vi "PH_uOPA_DelayController.PC _Settings.vi"(0 "VI in":refnum<vi>, 1 "serviceName":string, 2 "Axis Settings":T1={"Sign change"=FALSE, "Width"=0.0, "Calibration"=0.0, "Unit"="Steps", "Motor Type"=enum."Unspecific", "Unit Width"="", "Unit CF"=""}, 4 "no link":bool, 5 "error in (no error)":errorcluster) -> (14 "VI out":refnum<vi>, 19 "error out":errorcluster)   [LabVIEW 2014, in "PH_uOPA_DelayController.lvlib"]
uses:
  PH_uOPA_DelayController.lvlib
  PH_Basics/PH_Stepmotor_BaseClass/PH_Stepmotor_BaseClass.Axis Settings.ctl
  PH_Basics/PH_Stepmotor_BaseClass/PH_Stepmotor_BaseClass.Motor Type.ctl
  PH_Basics/PH_AxisGUI_BaseClass/PH_AxisGUI_BaseClass.lvlib
  PH_Basics/PH_Stepmotor_BaseClass/PH_Stepmotor_BaseClass.lvlib
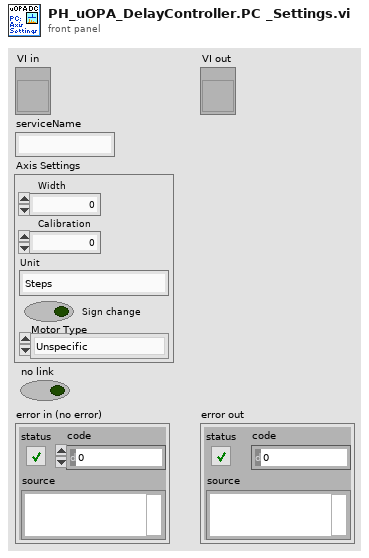
[diagram p1: front panel]
types:
  T1 = typedef "PH_Stepmotor_BaseClass.lvlib/PH_Stepmotor_BaseClass.Axis Settings.ctl" = cluster{"Sign change":bool, "Width":dbl, "Calibration":dbl, "Unit":string, "Motor Type":T2, "Unit Width":string, "Unit CF":string}
  T2 = typedef "PH_Stepmotor_BaseClass.lvlib/PH_Stepmotor_BaseClass.Motor Type.ctl" = enum16{"Unspecific", "OWIS 49.120.2633", "OWIS 49.060.1033", "OWIS 43.040.2558", "Diamond Motion 2200 series", "OWIS 49.120.266B.MV6", "Calorimeter", "Linear Stage 1", "MICOS VT-80", "MICOS VT-80 S", "Standa Rotstage nt0.95A", "PUF RA 320.200", "PUF RA 800.200", "PUF RA 800.400", "PUF RA 400.50", "1324.nn.800.50", "1324.n9c.800.50", "1324.nn.320.200", "1324.nn.400.200", "1324.nn.800.200", "1324.nn.400.50", "1324.8c9c.800.50", "1324.8c9c.400.200"}
  T3 = typedef "PH_uOPA_DelayController.lvlib/PH_uOPA_DelayController.i attribute.ctl" = cluster{"GUI Refs":cluster{"Current Pump Peak":refnum<vi>, "Current uOPA Peak":refnum<vi>, "Pump Peak":refnum<vi>, "uOPA Peak":refnum<vi>, "uOPA Target":refnum<vi>, "uOPA Limits [%]":refnum<vi>, "sample length":refnum<vi>, "Pump Target":refnum<vi>, "Pump Limit":refnum<vi>, "Pump running":refnum<vi>, "Feedback Control":refnum<vi>, "Control Status":refnum<vi>, "uOPA Mean":refnum<vi>, "Current uOPA Mean":refnum<vi>}, "uOPA Target":dbl, "uOPA Limits [%]":T4, "Sample Length":i32, "Initialize Mean":bool, "Pump Target":dbl, "Pump Limit [%]":dbl, "Feedback Control":bool, "Control Status":T5, "last Mean":dbl, "last direction":T6, "Axis Settings":T1, "Width while feedback":dbl}
  T4 = typedef "PH_uOPA_DelayController.lvlib/PH_uOPA_DelayController.Limit.ctl" = cluster{"low":dbl, "activate":dbl, "fine":dbl}
  T5 = typedef "PH_uOPA_DelayController.lvlib/PH_uOPA_DelayController.Control Status.ctl" = enum32{"off", "Pump off", "calculating", "too low", "activated", "fine"}
  T6 = typedef "PH_Stepmotor_BaseClass.lvlib/PH_Stepmotor_BaseClass.Axis Direction.ctl" = enum16{"forward", "backward"}
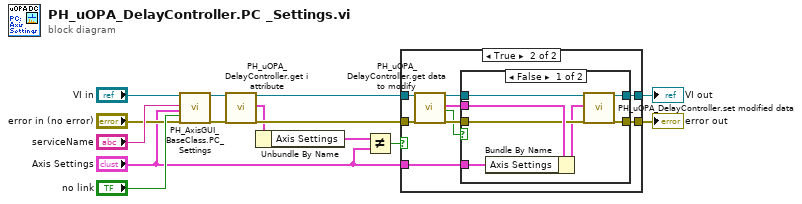
[diagram p0: block diagram]
diagram:
  n1 = call "PH_AxisGUI_BaseClass.PC_Settings.vi"("i ref in"="VI in", "Service Name"="serviceName", "Axis Settings"="Axis Settings", "No Link?"="no link", "error in"="error in (no error)") -> ("i ref out"=w6:refnum<vi>, "error"=w10:errorcluster)  [unwired: 12 in, 1 out]
  n2 = call "PH_uOPA_DelayController.get i attribute.vi"("i ref in"=w6, "error in (no error)"=w10) -> ("i ref out"=w5:refnum<vi>, "i attribute"=w4:T3, "error out"=w7:errorcluster)  [unwired: 15 in]
  n3 = Unbundle By Name(w4) -> ("Axis Settings"=w3:T1)
  n4 = Not Equal?(x=w3, y="Axis Settings") -> (x != y?=w1:bool)
  n5 = case shown="True" w1 {
    tunnel: [w16 w24] -> w14
    tunnel: w5 -> [w16 w22]
    tunnel: [w15 w21] -> w13
    tunnel: w7 -> [w15 w19]
    tunnel: "Axis Settings" -> [_ w18]
    frame False {
    }
    frame True {
      n6 = call "PH_uOPA_DelayController.get data to modify.vi"("i ref in"=w22, "error in (no error)"=w19) -> ("i ref out"=w23:refnum<vi>, "i attribute"=w25:T3, "timed out"=w17:bool, "error out"=w20:errorcluster)  [unwired: 14 in]
      n7 = case shown="False" w17 {
        tunnel: w25 -> [w32 _]
        tunnel: [w31 w34] -> w24
        tunnel: w23 -> [w30 w34]
        tunnel: [w29 w33] -> w21
        tunnel: w20 -> [w28 w33]
        tunnel: w18 -> [w26 _]
        frame False {
          n8 = Bundle By Name(cluster=w32, "Axis Settings"=w26) -> (w27:T3)
          n9 = call "PH_uOPA_DelayController.set modified data.vi"("i ref in"=w30, "i attribute"=w27, "error in (no error)"=w28) -> ("i ref out"=w31:refnum<vi>, "error out"=w29:errorcluster)  [unwired: 15 in]
        }
        frame True {
        }
      }
    }
  }
  "VI out" <- w14
  "error out" <- w13
